vi "read top level item.vi"(11 "Builder in":refnum<class "Builder.lvclass">) -> (2 "top level item":string)   [LabVIEW 2024, in "Builder.lvclass"]
uses:
  Builder.lvclass
  Builder.lvclass/Builder.ctl
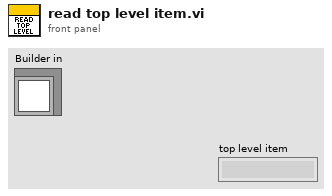
[diagram p1: front panel]
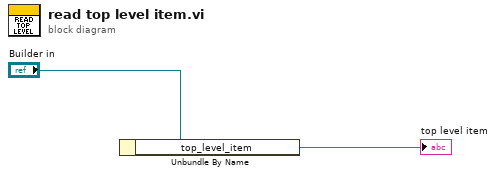
[diagram p0: block diagram]
diagram:
  n1 = Unbundle By Name("Builder in") -> ("top_level_item"=→"top level item":string)
